vi "Algae Controller.vi"(8 "error in":errorcluster) -> ()   [LabVIEW 2023]
doc: "This VI executes continuously carrying out the current operation and responding to updates or new operations. It will often contain the timing or control code that is difficult to place directly in TeleOp. This VI generally opens all sensors and motors and isolates the rest of the robot code from knowing how the operations are carried out."
uses:
  <vilib>/Rock Robotics/WPI/Framework/Completion Status.ctl
  Algae Setpoints.ctl
  Algae Operations.ctl
  Support Code/Teleop Util/Algae States.ctl
  <vilib>/Rock Robotics/WPI/ThirdParty/REV Robotics/REVLib/Typedef/Spark MAX Idle Mode.ctl
  <vilib>/Rock Robotics/WPI/ThirdParty/REV Robotics/REVLib/Typedef/Spark MAX Control Type.ctl
  <vilib>/Rock Robotics/WPI/ThirdParty/REV Robotics/REVLib/SubVI/Public/SPARK Open Brushless.vi
  <vilib>/Rock Robotics/WPI/ThirdParty/REV Robotics/REVLib/SubVI/Public/SPARK Configure Basic Idle Mode.vi
  <vilib>/Rock Robotics/WPI/ThirdParty/REV Robotics/REVLib/SubVI/Public/SPARK Configure Power Smart Current Limit.vi
  <vilib>/Rock Robotics/WPI/ThirdParty/REV Robotics/REVLib/SubVI/Public/SPARK Configure Soft Limit Forward.vi
  <vilib>/Rock Robotics/WPI/ThirdParty/REV Robotics/REVLib/SubVI/Public/SPARK Configure Soft Limit Reverse.vi
  <vilib>/Rock Robotics/WPI/ThirdParty/REV Robotics/REVLib/SubVI/Public/SPARK Get Encoder Status Position.vi
  <vilib>/Rock Robotics/Network Tables/NT Write String.vi
  <vilib>/Rock Robotics/WPI/ThirdParty/REV Robotics/REVLib/SubVI/Public/SPARK Get Device Status Output Current.vi
  Framework/Robot Global Data.vi
  <vilib>/Rock Robotics/Network Tables/NT Write Boolean.vi
panel:
  out "Waveform Chart":dbl(graph)=0.1325334757566452
  in  "PID Constants":T1={"P Gain"=0.08, "I Gain"=0.0, "D Gain"=0.0, "F Gain"=0.0, "I Zone"=0.002, "Min Output"=-0.8, "Max Output"=0.8}
  in  "Interactive Values":T2={"Operation"=enum."Reserve", "Setpoint"=0.0, "Duration"=0.0, "Algae State"=enum."Intake Algae", "Negate or Confirm?"=FALSE}
  out "Current\nCmd":string="Started at  16:44:38.557\n: Immediate,  S 0.0, D 0.000000"
  in  "Buttons":cluster{"Execute Cmd":bool, "Abort Cmd":bool}
  out "Command Timing":cluster{"Start Time (ms)":u32, "Iterations":i32}={"Start Time (ms)"=1128151, "Iterations"=0}
  out "Status":T5=enum."Incomplete"
  # "Tip: It may be helpful to observe inputs and sensor values.\nYou may also want to display tuning or debugging controls."
  # "Interactive Command: You may fill in the settings for a command\nand schedule it with the Execute button. You can observe and abort\nany command while fine tuning the code for the controller."
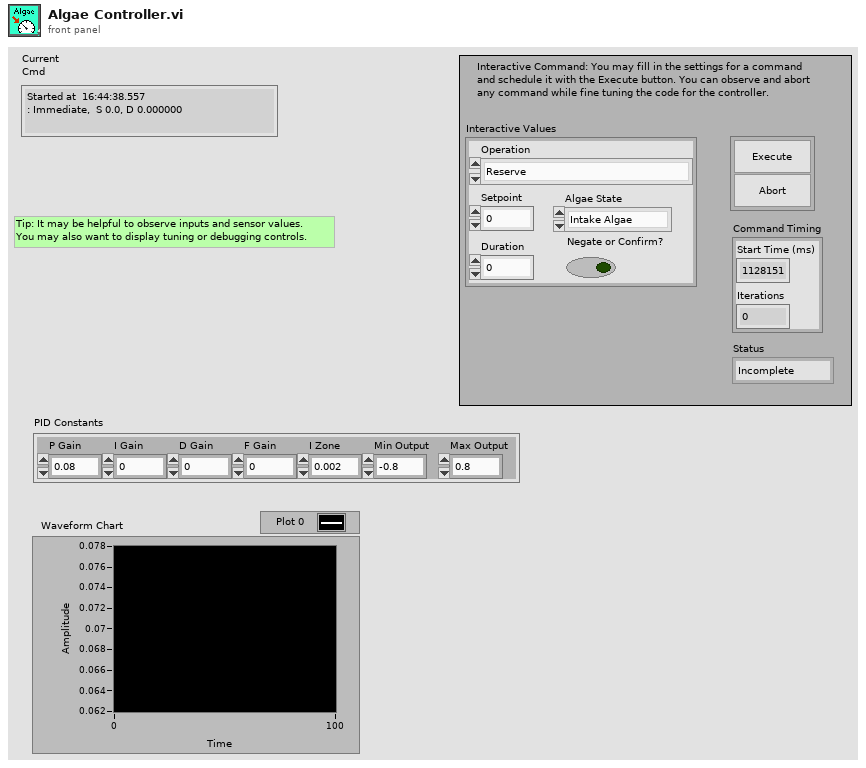
[diagram p1: front panel]
types:
  T1 = cluster{"P Gain":dbl, "I Gain":dbl, "D Gain":dbl, "F Gain":dbl, "I Zone":dbl, "Min Output":dbl, "Max Output":dbl}
  T2 = typedef "Algae Setpoints.ctl" = cluster{"Operation":T3, "Setpoint":dbl, "Duration":dbl, "Algae State":T4, "Negate or Confirm?":bool}
  T3 = typedef "Algae Operations.ctl" = enum16{"Reserve", "Read Current", "Immediate", "Calibrate"}
  T4 = typedef "Algae States.ctl" = enum16{"Idle", "Intake Algae", "Outtake Algae", "Stow", "Manual Overrides"}
  T5 = typedef "Completion Status.ctl" = enum16{"Successful", "Aborted", "Incomplete"}
  T6 = typedef "Spark MAX Idle Mode.ctl" = enum16{"Coast", "Brake"}
  T7 = typedef "WPI_MotorControlDeviceRef.ctl" = cluster{"DeviceStatus":errorcluster, "Type":T8, "PWM":cluster{"PWM Channel":T9, "DeadBand":T10}, "CAN":cluster{"Device Number":u8, "SetOutput VI Ref":variant, "GetOutput VI Ref":variant, "Enable VI Ref":variant, "Disable VI Ref":variant, "Data":variant}, "Invert":bool, "DIO PWM":cluster{"PWM \"Enable\" Channel":T9, "DIOChannel":T11, "PWM Rate":dbl}}
  T8 = typedef "WPI_MotorControlType.ctl" = enum16{"PWM", "CAN", "DIO PWM"}
  T9 = typedef "FPGA_DIOPWMChannel.ctl" = enum8{"PWM 0", "PWM 1", "PWM 2", "PWM 3", "PWM 4", "PWM 5", "PWM 6", "PWM 7", "PWM 8", "PWM 9", "PWM MXP 0", "PWM MXP 1", "PWM MXP 2", "PWM MXP 3", "PWM MXP 4", "PWM MXP 5", "PWM MXP 6", "PWM MXP 7", "PWM MXP 8", "PWM MXP 9", "Invalid"}
  T10 = typedef "WPI_PWMDeadband.ctl" = cluster{"Name":string, "maxPositivePwm":i32, "minPositivePwm":i32, "centerPwm":i32, "maxNegativePwm":i32, "minNegativePwm":i32, "angularRange":u16}
  T11 = typedef "FPGA_DIOChannel.ctl" = enum8{"DIO 0", "DIO 1", "DIO 2", "DIO 3", "DIO 4", "DIO 5", "DIO 6", "DIO 7", "DIO 8", "DIO 9", "DIO MXP 0", "DIO MXP 1", "DIO MXP 2", "DIO MXP 3", "DIO MXP 4", "DIO MXP 5", "DIO MXP 6", "DIO MXP 7", "DIO MXP 8", "DIO MXP 9", "DIO MXP 10", "DIO MXP 11", "DIO MXP 12", "DIO MXP 13", "DIO MXP 14", "DIO MXP 15", "SPI Port CS1", "SPI Port CS2", "SPI Port CS3", "SPI Port MISO", "SPI Port MOSI", "Invalid"}
  T12 = typedef "Command Status Info.ctl" = cluster{"Name":string, "Status":T5, "notifier out":T13}
  T13 = typedef "Completion Notifier.ctl" = refnum<notifier>
  T14 = cluster{"Current Command":T2, "Command Timing":cluster{"Start Time (ms)":u32, "Iterations":i32}, "Command Arguments":cluster{"Command Info":T12, "Description":string, "Default Command":T2, "queue out":refnum<queue>, "Subsystem Name":string}}
  T15 = typedef "Spark MAX Control Type.ctl" = enum16{"Percent VBus", "Voltage", "Velocity", "Position", "Smart Motion", "Current", "Smart Velocity", "MAXMotion Position", "MAXMotion Velocity"}
  T16 = typedef "Algae Setpoint.ctl" = enum16{"Idle", "Stow", "Intake/Outtake"}
  T17 = cluster{"Setpoint Configs":cluster{"Position Setpoint":dbl, "Algae State":T16, "Power Output":dbl}[]}
  T18 = cluster{"Position Setpoint":dbl, "Algae State":T16, "Power Output":dbl}[]
  T19 = cluster{"Position Setpoint":dbl, "Algae State":T16, "Power Output":dbl}
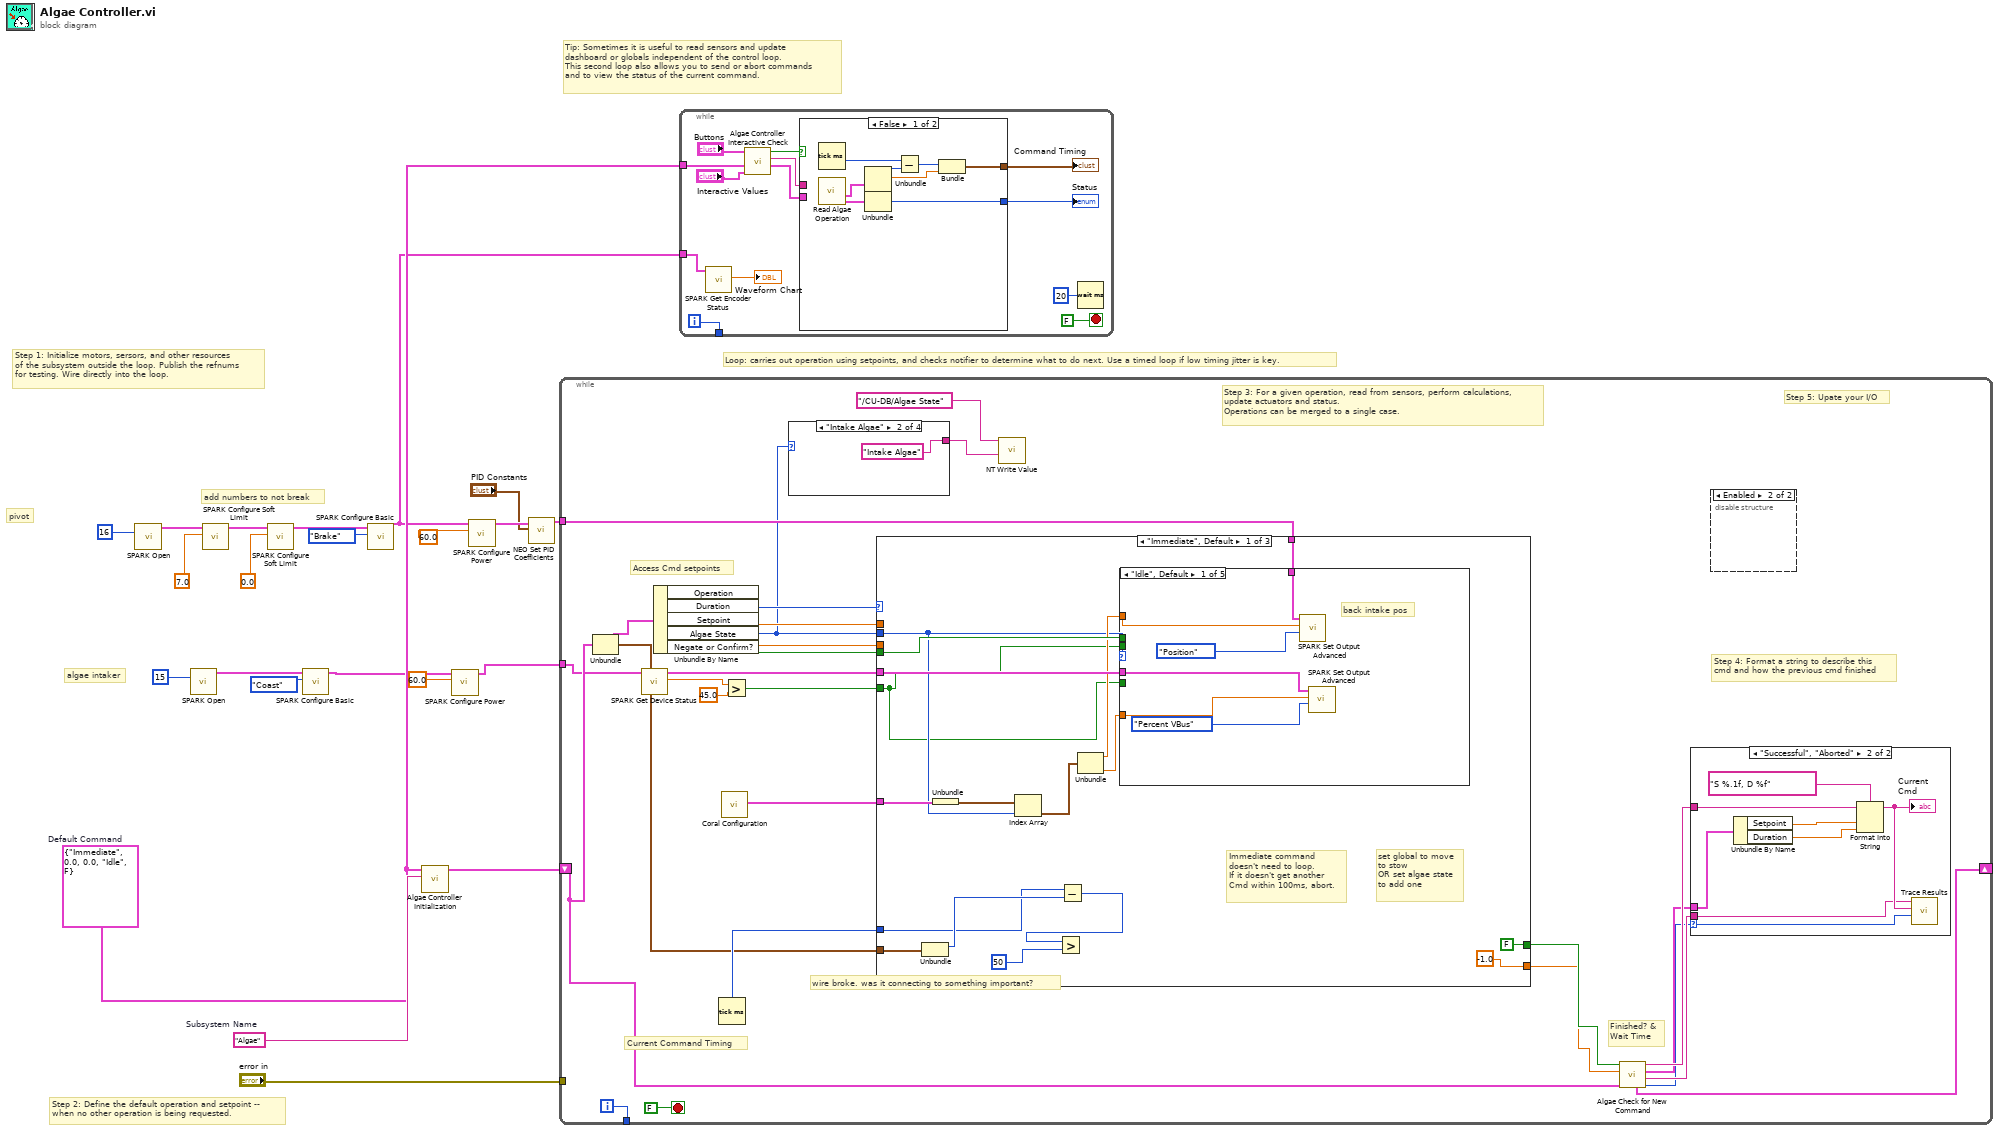
[diagram p0: block diagram]
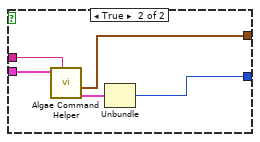
[diagram p2: hidden frame]
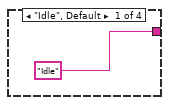
[diagram p3: hidden frame]
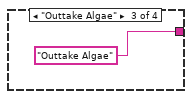
[diagram p4: hidden frame]
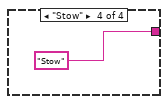
[diagram p5: hidden frame]
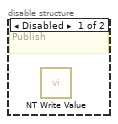
[diagram p6: hidden frame]
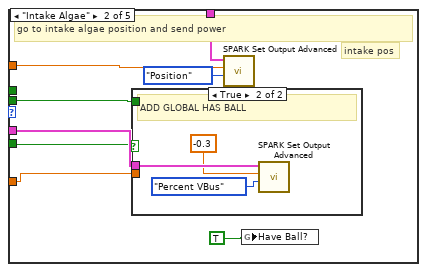
[diagram p8: hidden frame]
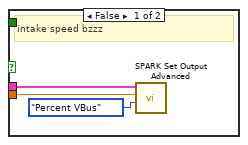
[diagram p9: hidden frame]
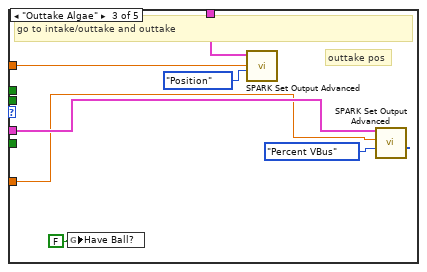
[diagram p10: hidden frame]
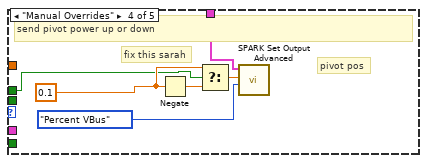
[diagram p11: hidden frame]
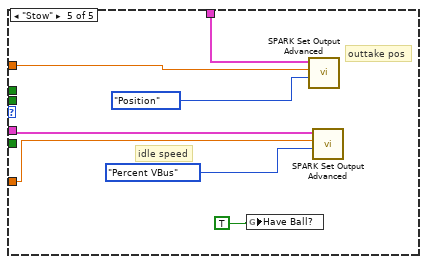
[diagram p12: hidden frame]
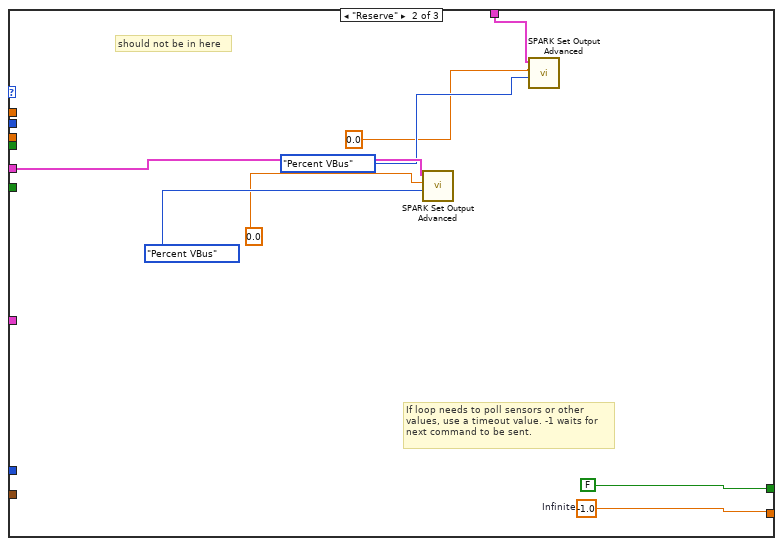
[diagram p13: hidden frame]
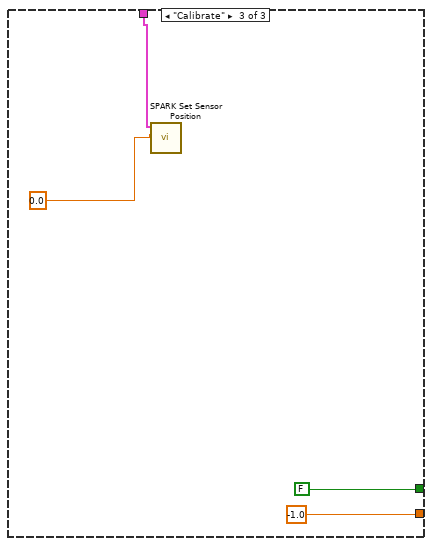
[diagram p14: hidden frame]
diagram:
  w19 = T2 {"Operation"=enum."Immediate", "Setpoint"=0.0, "Duration"=0.0, "Algae State"=enum."Idle", "Negate or Confirm?"=FALSE}  # Default Command
  w20 = "Algae"  # Subsystem Name
  # "add numbers to not break"
  # "algae intaker"
  # "pivot"
  # "Tip: Sometimes it is useful to read sensors and update\ndashboard or globals independent of the control loop.\nThis second loop also allows you to send or abort commands\nand to view the status of the current command."
  # "Step 2: Define the default operation and setpoint --\nwhen no other operation is being requested."
  # "Step 1: Initialize motors, sersors, and other resources\nof the subsystem outside the loop. Publish the refnums\nfor testing. Wire directly into the loop."
  # "Loop: carries out operation using setpoints, and checks notifier to determine what to do next. Use a timed loop if low timing jitter is key."
  n1 = call-poly <vilib>:"SPARK Open.vi"("Device Number"=u8 16) -> ("MotorControlDeviceRef"=w16:T7)  [unwired: 9 in, 1 out]
  n2 = call-poly <vilib>:"SPARK Open.vi"("Device Number"=u8 15) -> ("MotorControlDeviceRef"=w14:T7)  [unwired: 9 in, 1 out]
  n3 = call-poly <vilib>:"SPARK Configure Soft Limit.vi"("Soft Limit"=7.0, "MotorControlDeviceRef in"=w16) -> ("MotorControlDeviceRef out"=w15:T7)  [unwired: 8 in, 1 out]
  n4 = call-poly <vilib>:"SPARK Configure Soft Limit.vi"("Soft Limit"=0.0, "MotorControlDeviceRef in"=w15) -> ("MotorControlDeviceRef out"=w13:T7)  [unwired: 8 in, 1 out]
  n5 = call-poly <vilib>:"SPARK Configure Basic.vi"("Idle Mode"=Spark_MAX_Idle_Mode."Coast", "MotorControlDeviceRef in"=w14) -> ("MotorControlDeviceRef out"=w10:T7)  [unwired: 8 in, 1 out]
  n6 = call-poly <vilib>:"SPARK Configure Basic.vi"("Idle Mode"=Spark_MAX_Idle_Mode."Brake", "MotorControlDeviceRef in"=w13) -> ("MotorControlDeviceRef out"=w4:T7)  [unwired: 8 in, 1 out]
  n7 = call "Algae Controller Initialization.vi"("Subsystem Name"=w20, "Default Command"=w19) -> ("Current Command"=w21:T14)  [unwired: 9 in]
  n8 = call-poly <vilib>:"SPARK Configure Power.vi"("Primay Current Limit (80A)"=60.0, "MotorControlDeviceRef in"=w10) -> ("MotorControlDeviceRef out"=w9:T7)  [unwired: 8 in, 1 out]
  n9 = call-poly <vilib>:"SPARK Configure Power.vi"("Primay Current Limit (80A)"=60.0, "MotorControlDeviceRef in"=w4) -> ("MotorControlDeviceRef out"=w3:T7)  [unwired: 8 in, 1 out]
  n10 = call "NEO Set PID Coefficients.vi"("PID Constants"="PID Constants", "MotorControlDeviceRef in"=w3) -> ("MotorControlDeviceRef out"=w2:T7)  [unwired: 6 in, 1 out]
  n11 = while {
    shift-right: [w42] -> _
    shift-left: w21 -> [w35]
    tunnel: [w48] -> _
    tunnel: "error in" -> [_]
    tunnel: w9 -> [w34]
    tunnel: w2 -> [w27]
    i -> [w48]
    stop <- FALSE stop-if-true
    # "wire broke. was it connecting to something important?"
    # "Step 5: Upate your I/O"
    # "Step 4: Format a string to describe this\ncmd and how the previous cmd finished"
    # "Current Command Timing"
    # "Access Cmd setpoints"
    # "Finished? &\nWait Time"
    # "Step 3: For a given operation, read from sensors, perform calculations,\nupdate actuators and status.\nOperations can be merged to a single case."
    n12 = Unbundle(w35) -> ("Current Command"=w47:T2, "Command Timing"=w44:cluster{"Start Time (ms)":u32, "Iterations":i32})  [unwired: 1 out]
    n13 = call-poly <vilib>:"SPARK Get Device Status.vi"("MotorControlDevRef in"=w34) -> ("Current"=w32:dbl, "MotorControlDevRef out"=w33:T7)  [unwired: 7 in, 2 out]
    n14 = Unbundle By Name(w47) -> ("Operation"=w26:T3, "Duration"=w46:dbl, "Setpoint"=w43:dbl, "Algae State"=w25:T4, "Negate or Confirm?"=w29:bool)
    n15 = Tick Count (ms)() -> (millisecond timer value=w45:u32)
    n16 = call "Coral Configuration.vi"() -> ("Algae Config"=w28:T17)  [unwired: 10 in, 1 out]
    n17 = Greater?(x=w32, y=45.0) -> (0:w30:bool)
    n18 = case shown="\"Intake Algae\"" w25 {
      tunnel: ["Idle" "Intake Algae" "Outtake Algae" "Stow"] -> w24
      frame "Idle", Default {
      }
      frame "Intake Algae" {
      }
      frame "Outtake Algae" {
      }
      frame "Stow" {
      }
    }
    n19 = case shown="\"Immediate\", Default" w26 {
      tunnel: [-1.0 ("Infinite") w126 -1.0 ("Infinite")] -> w40
      tunnel: [FALSE ("ignore previous (F)") FALSE ("ignore previous (F)") FALSE ("ignore previous (F)")] -> w41
      tunnel: w44 -> [w75 _ _]
      tunnel: w46 -> [_ _ _]
      tunnel: w45 -> [w74 _ _]
      tunnel: w43 -> [_ _ _]
      tunnel: w25 -> [w64 _ _]
      tunnel: w27 -> [w72 w120 w130]
      tunnel: w33 -> [w71 w124 _]
      tunnel: w30 -> [w63 _ _]
      tunnel: w29 -> [w66 _ _]
      tunnel: w28 -> [w70 _ _]
      frame "Immediate", Default {
        # "set global to move\nto stow\nOR set algae state \nto add one"
        # "Immediate command\ndoesn't need to loop.\nIf it doesn't get another\nCmd within 100ms, abort."
        n20 = Unbundle(w75) -> ("Start Time (ms)"=w78:u32)  [unwired: 1 out]
        n21 = Unbundle(w70) -> ("Setpoint Configs"=w69:T18)
        n22 = Index Array(array=w69, index=w64) -> (element=w68:T19)
        n23 = Subtract(x=w74, y=w78) -> (x-y=w77:u32)
        n24 = Greater?(x=w77, y=u8 50 ("Left Motor")) -> ()  [unwired: 1 out]
        n25 = Unbundle(w68) -> ("Position Setpoint"=w65:dbl, "Power Output"=w67:dbl)  [unwired: 1 out]
        n26 = case shown="\"Idle\", Default" w64 {
          tunnel: w72 -> [w83 w92 w104 w111 w116]
          tunnel: w71 -> [w81 w91 w101 _ w117]
          tunnel: w63 -> [_ w89 _ _ _]
          tunnel: w67 -> [w79 w88 w100 _ w114]
          tunnel: w65 -> [w80 w87 w102 _ w113]
          tunnel: w66 -> [_ _ _ w106 _]
          tunnel: w63 -> [_ w86 _ _ _]
          frame "Idle", Default {
            # "back intake pos"
            n27 = call <vilib>:"SPARK Set Output Advanced.vi"("Control Mode"=Spark_MAX_Control_Type."Position", "Setpoint"=w80, "MotorControlDevRef"=w83) -> ()  [unwired: 7 in, 2 out]
            n28 = call <vilib>:"SPARK Set Output Advanced.vi"("Control Mode"=Spark_MAX_Control_Type."Percent VBus", "Setpoint"=w79, "MotorControlDevRef"=w81) -> ()  [unwired: 7 in, 2 out]
          }
          frame "Intake Algae" {
            # "intake pos"
            # "go to intake algae position and send power"
            n29 = case shown="True" w89 {
              tunnel: w91 -> [w94 w98]
              tunnel: w88 -> [w93 _]
              tunnel: w86 -> [_ _]
              frame False {
                # "intake speed bzzz"
                n30 = call <vilib>:"SPARK Set Output Advanced.vi"("Control Mode"=Spark_MAX_Control_Type."Percent VBus", "Setpoint"=w93, "MotorControlDevRef"=w94) -> ()  [unwired: 7 in, 2 out]
              }
              frame True {
                # "ADD GLOBAL HAS BALL"
                n31 = call <vilib>:"SPARK Set Output Advanced.vi"("Control Mode"=Spark_MAX_Control_Type."Percent VBus", "Setpoint"=-0.3, "MotorControlDevRef"=w98) -> ()  [unwired: 7 in, 2 out]
              }
            }
            n32 = call <vilib>:"SPARK Set Output Advanced.vi"("Control Mode"=Spark_MAX_Control_Type."Position", "Setpoint"=w87, "MotorControlDevRef"=w92) -> ()  [unwired: 7 in, 2 out]
            n33 = global write "Robot Global Data.vi" "Have Ball?"(TRUE ("Have Ball?")) -> ()
          }
          frame "Outtake Algae" {
            # "outtake pos"
            # "go to intake/outtake and outtake"
            n34 = global write "Robot Global Data.vi" "Have Ball?"(FALSE ("Have Ball?")) -> ()
            n35 = call <vilib>:"SPARK Set Output Advanced.vi"("Control Mode"=Spark_MAX_Control_Type."Position", "Setpoint"=w102, "MotorControlDevRef"=w104) -> ()  [unwired: 7 in, 2 out]
            n36 = call <vilib>:"SPARK Set Output Advanced.vi"("Control Mode"=Spark_MAX_Control_Type."Percent VBus", "Setpoint"=w100, "MotorControlDevRef"=w101) -> ()  [unwired: 7 in, 2 out]
          }
          frame "Manual Overrides" {
            w107 = 0.1 ("Setpoint")
            # "fix this sarah"
            # "pivot pos"
            # "send pivot power up or down"
            n37 = Negate(x=w107) -> (-x=w109:dbl)
            n38 = Select(t=w107, s=w106, f=w109) -> (s? t:f=w108:dbl)
            n39 = call <vilib>:"SPARK Set Output Advanced.vi"("Control Mode"=Spark_MAX_Control_Type."Percent VBus", "Setpoint"=w108, "MotorControlDevRef"=w111) -> ()  [unwired: 7 in, 2 out]
          }
          frame "Stow" {
            # "outtake pos"
            # "idle speed"
            n40 = global write "Robot Global Data.vi" "Have Ball?"(TRUE ("Have Ball?")) -> ()
            n41 = call <vilib>:"SPARK Set Output Advanced.vi"("Control Mode"=Spark_MAX_Control_Type."Position", "Setpoint"=w113, "MotorControlDevRef"=w116) -> ()  [unwired: 7 in, 2 out]
            n42 = call <vilib>:"SPARK Set Output Advanced.vi"("Control Mode"=Spark_MAX_Control_Type."Percent VBus", "Setpoint"=w114, "MotorControlDevRef"=w117) -> ()  [unwired: 7 in, 2 out]
          }
        }
      }
      frame "Reserve" {
        w126 = -1.0  # Infinite
        # "should not be in here"
        # "If loop needs to poll sensors or other\nvalues, use a timeout value. -1 waits for\nnext command to be sent."
        n43 = call <vilib>:"SPARK Set Output Advanced.vi"("Control Mode"=Spark_MAX_Control_Type."Percent VBus", "Setpoint"=0.0, "MotorControlDevRef"=w124) -> ()  [unwired: 7 in, 2 out]
        n44 = call <vilib>:"SPARK Set Output Advanced.vi"("Control Mode"=Spark_MAX_Control_Type."Percent VBus", "Setpoint"=0.0, "MotorControlDevRef"=w120) -> ()  [unwired: 7 in, 2 out]
      }
      frame "Calibrate" {
        n45 = call <vilib>:"SPARK Set Sensor Position.vi"("Position"=0.0, "MotorControlDeviceRef"=w130) -> ()  [unwired: 8 in, 2 out]
      }
    }
    n46 = call-poly <vilib>:"NT Write Value.vi"("value"=w24, "name"="/CU-DB/Algae State") -> ()  [unwired: 9 in, 1 out]
    n47 = call "Algae Check for New Command.vi"("Current Command"=w35, "Wait time (ms)"=w40, "Finished?"=w41) -> ("Completion"=w36:T5, "Subsystem Name"=w37:string, "Current Command"=w38:T2, "Initial Trace String"=w39:string, "NextCommand"=w42:T14)  [unwired: 4 in]
    n48 = case shown="\"Successful\", \"Aborted\"" w36 {
      selector: w36 -> [_ w61]
      tunnel: w39 -> [_ w57]
      tunnel: w38 -> [_ w58]
      tunnel: w37 -> [_ w54]
      frame "Incomplete", Default {
        # "Continuing current command"
      }
      frame "Successful", "Aborted" {
        # "Report and setup for next command"
        n49 = Unbundle By Name(w58) -> ("Setpoint"=w60:dbl, "Duration"=w55:dbl)
        n50 = Format Into String(format string="S %.1f, D %f", initial string=w57, w60, w55) -> (resulting string=w56:string)  [unwired: 1 in, 1 out]
        "Current\nCmd" <- w56
        n51 = call <vilib>:"Trace Results.vi"("Status of previous command"=w61, "Description"=w56, "Subsystem"=w54) -> ()  [unwired: 9 in]
      }
    }
    n52 = disable-structure shown="Enabled" {
      frame Disabled {
        # "Publish"
        n53 = call-poly <vilib>:"NT Write Value.vi"() -> ()  [unwired: 11 in, 1 out]
      }
      frame Enabled {
      }
    }
  }
  n54 = while {
    tunnel: w19 -> [w140]
    tunnel: w4 -> [w132]
    tunnel: [w131] -> _
    i -> [w131]
    stop <- FALSE stop-if-true
    n55 = call-poly <vilib>:"SPARK Get Encoder Status.vi"("MotorControlDevRef in"=w132) -> ("Sensor Position"=→"Waveform Chart":dbl)  [unwired: 7 in, 3 out]
    n56 = call "Algae Controller Interactive Check.vi"("Interactive Command in"="Interactive Values", "Default Command"=w140, "Buttons"="Buttons") -> ("Interactive Command out"=w137:T2, "Trace String"=w138:string, "Schedule"=w139:bool)  [unwired: 6 in]
    n57 = case shown="False" w139 {
      tunnel: [w151 w156] -> w136
      tunnel: w137 -> [_ w154]
      tunnel: [w147 w152] -> w135
      tunnel: w138 -> [_ w155]
      frame False {
        n58 = Tick Count (ms)() -> (millisecond timer value=w146:u32)
        n59 = call "Read Algae Operation.vi"() -> ("Command Info"=w144:T12, "SubSystem Data"=w145:T2)  [unwired: 9 in, 1 out]
        n60 = Unbundle(w145) -> ("Operation"=w150:T3, "Setpoint"=w148:dbl)  [unwired: 3 out]
        n61 = Unbundle(w144) -> ("Status"=w151:T5)  [unwired: 2 out]
        n62 = Subtract(x=w146, y=w150) -> (x-y=w149:u32)
        n63 = Bundle(w149, "Setpoint"=w148) -> (w147:cluster{u32, "Setpoint":dbl})  [unwired: 1 in]
      }
      frame True {
        n64 = call "Algae Command Helper.vi"("Description"=w155, "SubSystem Data"=w154) -> ("Command Info Out"=w153:T12, "Command Timing"=w152:cluster{"Start Time (ms)":u32, "Iterations":i32})  [unwired: 7 in, 1 out]
        n65 = Unbundle(w153) -> ("Status"=w156:T5)  [unwired: 2 out]
      }
    }
    "Status" <- w136
    "Command Timing" <- w135
    n66 = Wait (ms)(milliseconds to wait=u32 20) -> ()  [unwired: 1 out]
  }
